vi "Configure Measurement Averaging.vi"(7 "Enable Average Mode (T: Enable)":bool=TRUE, 8 "error in (no error)":errorcluster, 9 "Averaging Mode (0: Exponential)":i32(ring) items=["Exponential", "Repeat"], 10 "Average Number (10)":i32=10 format="%.0g", 11 "VISA resource name":refnum<visa-resource-name>) -> (0 "error out":errorcluster, 3 "VISA resource name out":refnum<visa-resource-name>)   [LabVIEW 2014, in "Agilent MXA Series.lvlib"]
doc: "Configures the measurement averaging."
uses:
  Agilent MXA Series.lvlib
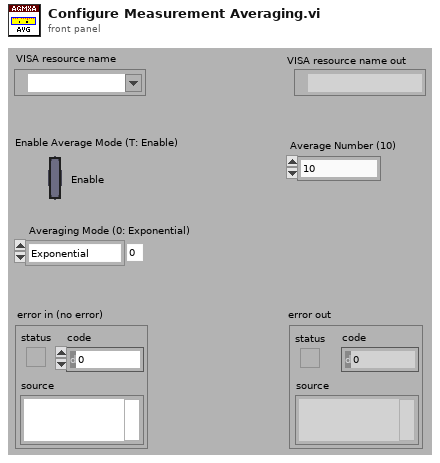
[diagram p1: front panel]
types:
  T1 = typedef "Agilent MXA Series.lvlib/Extended User Data.ctl" = cluster{"Measurement Type":i32, "Agilent MXA/EXA Model":i32}
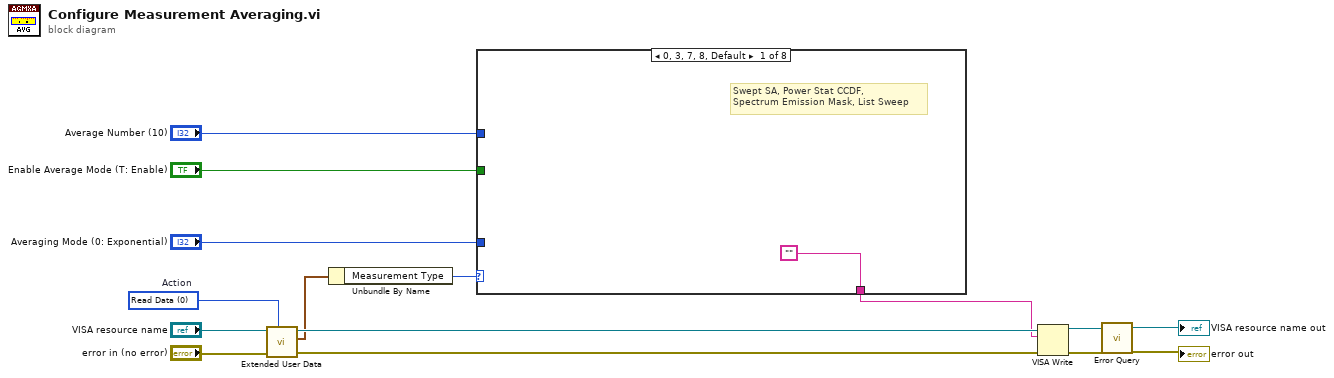
[diagram p0: block diagram]
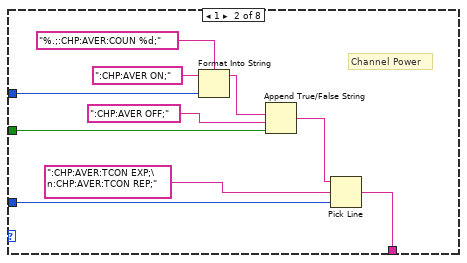
[diagram p2: hidden frame]
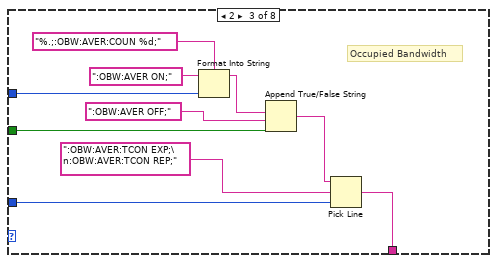
[diagram p3: hidden frame]
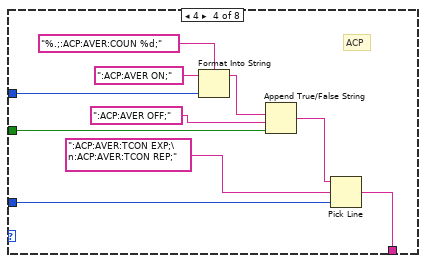
[diagram p4: hidden frame]
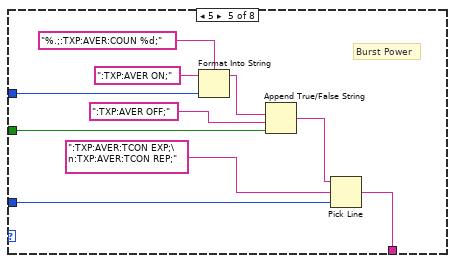
[diagram p5: hidden frame]
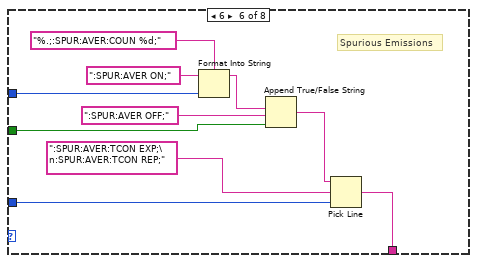
[diagram p6: hidden frame]
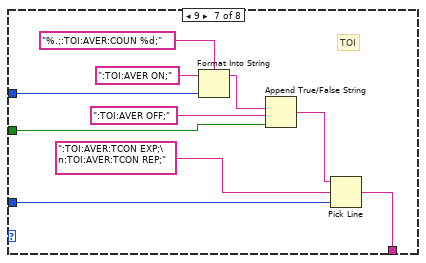
[diagram p7: hidden frame]
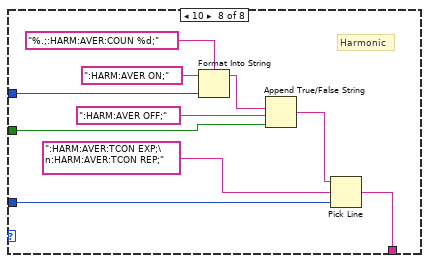
[diagram p8: hidden frame]
diagram:
  w7 = 0 items=["Read Data", "Write Data", "Clear Data", "Clear ALL Data"]  # Action
  n1 = call "Extended User Data.vi"("Action (1:Write Data)"=w7, "Error In (no error)"="error in (no error)", "VISA resource name in"="VISA resource name") -> ("Error Out"=w10:errorcluster, "User Data Out"=w6:T1, "VISA resource name out"=w11:refnum<visa-resource-name>)  [unwired: 6 in]
  n2 = Unbundle By Name(w6) -> ("Measurement Type"=w5:i32)
  n3 = case shown="0, 3, 7, 8, Default" w5 {
    tunnel: "Average Number (10)" -> [_ w26 w36 w46 w56 w66 w76 w86]
    tunnel: "Averaging Mode (0: Exponential)" -> [_ w24 w34 w44 w54 w64 w74 w84]
    tunnel: ["" w22 w32 w42 w52 w62 w72 w82] -> w1
    tunnel: "Enable Average Mode (T: Enable)" -> [_ w17 w27 w37 w47 w57 w67 w77]
    frame 0, 3, 7, 8, Default {
      # "Swept SA, Power Stat CCDF,\nSpectrum Emission Mask, List Sweep"
    }
    frame 1 {
      # "Channel Power"
      n4 = Format Into String(format string="%.;:CHP:AVER:COUN %d;", initial string=":CHP:AVER ON;", w26) -> (resulting string=w20:string)  [unwired: 1 in, 1 out]
      n5 = Append True/False String(1:w17, 2:":CHP:AVER OFF;" ("false string"), 3:w20) -> (0:w18:string)  [unwired: 1 in]
      n6 = Pick Line(string ("")=w18, multi-line string=":CHP:AVER:TCON EXP;\n:CHP:AVER:TCON REP;", line index=w24) -> (output string=w22:string)
    }
    frame 2 {
      # "Occupied Bandwidth"
      n7 = Format Into String(format string="%.;:OBW:AVER:COUN %d;", initial string=":OBW:AVER ON;", w36) -> (resulting string=w30:string)  [unwired: 1 in, 1 out]
      n8 = Append True/False String(1:w27, 2:":OBW:AVER OFF;" ("false string"), 3:w30) -> (0:w28:string)  [unwired: 1 in]
      n9 = Pick Line(string ("")=w28, multi-line string=":OBW:AVER:TCON EXP;\n:OBW:AVER:TCON REP;", line index=w34) -> (output string=w32:string)
    }
    frame 4 {
      # "ACP"
      n10 = Format Into String(format string="%.;:ACP:AVER:COUN %d;", initial string=":ACP:AVER ON;", w46) -> (resulting string=w40:string)  [unwired: 1 in, 1 out]
      n11 = Append True/False String(1:w37, 2:":ACP:AVER OFF;" ("false string"), 3:w40) -> (0:w38:string)  [unwired: 1 in]
      n12 = Pick Line(string ("")=w38, multi-line string=":ACP:AVER:TCON EXP;\n:ACP:AVER:TCON REP;", line index=w44) -> (output string=w42:string)
    }
    frame 5 {
      # "Burst Power"
      n13 = Format Into String(format string="%.;:TXP:AVER:COUN %d;", initial string=":TXP:AVER ON;", w56) -> (resulting string=w50:string)  [unwired: 1 in, 1 out]
      n14 = Append True/False String(1:w47, 2:":TXP:AVER OFF;" ("false string"), 3:w50) -> (0:w48:string)  [unwired: 1 in]
      n15 = Pick Line(string ("")=w48, multi-line string=":TXP:AVER:TCON EXP;\n:TXP:AVER:TCON REP;", line index=w54) -> (output string=w52:string)
    }
    frame 6 {
      # "Spurious Emissions"
      n16 = Format Into String(format string="%.;:SPUR:AVER:COUN %d;", initial string=":SPUR:AVER ON;", w66) -> (resulting string=w60:string)  [unwired: 1 in, 1 out]
      n17 = Append True/False String(1:w57, 2:":SPUR:AVER OFF;" ("false string"), 3:w60) -> (0:w58:string)  [unwired: 1 in]
      n18 = Pick Line(string ("")=w58, multi-line string=":SPUR:AVER:TCON EXP;\n:SPUR:AVER:TCON REP;", line index=w64) -> (output string=w62:string)
    }
    frame 9 {
      # "TOI"
      n19 = Format Into String(format string="%.;:TOI:AVER:COUN %d;", initial string=":TOI:AVER ON;", w76) -> (resulting string=w70:string)  [unwired: 1 in, 1 out]
      n20 = Append True/False String(1:w67, 2:":TOI:AVER OFF;" ("false string"), 3:w70) -> (0:w68:string)  [unwired: 1 in]
      n21 = Pick Line(string ("")=w68, multi-line string=":TOI:AVER:TCON EXP;\n:TOI:AVER:TCON REP;", line index=w74) -> (output string=w72:string)
    }
    frame 10 {
      # "Harmonic"
      n22 = Format Into String(format string="%.;:HARM:AVER:COUN %d;", initial string=":HARM:AVER ON;", w86) -> (resulting string=w80:string)  [unwired: 1 in, 1 out]
      n23 = Append True/False String(1:w77, 2:":HARM:AVER OFF;" ("false string"), 3:w80) -> (0:w78:string)  [unwired: 1 in]
      n24 = Pick Line(string ("")=w78, multi-line string=":HARM:AVER:TCON EXP;\n:HARM:AVER:TCON REP;", line index=w84) -> (output string=w82:string)
    }
  }
  n25 = VISA Write(VISA resource name=w11, write buffer=w1, error in (no error)=w10) -> (VISA resource name out=w12:refnum<visa-resource-name>, error out=w13:errorcluster)  [unwired: 1 out]
  n26 = call "Error Query.vi"("error in (no error)"=w13, "VISA resource name"=w12) -> ("error out"=→"error out":errorcluster, "VISA resource name out"=→"VISA resource name out":refnum<visa-resource-name>)  [unwired: 6 in, 2 out]
